vi "SPCCreateSetUpAsciiString.vi"(10 "Value":string[](array[string])=["5.0033574e-08"], 11 "Key":string[](array[string])=["SP_TAC_R,F,"]) -> (3 "SetUpAsciiString":string)   [LabVIEW 2019]
doc: "This VI demonstrates how specific parameters can be entered into an ASCII SetUp-block replacing their default values.\nProvide the Key up to and including the format specifier and trailing comma.\n\ninfo@becker-hickl.com"
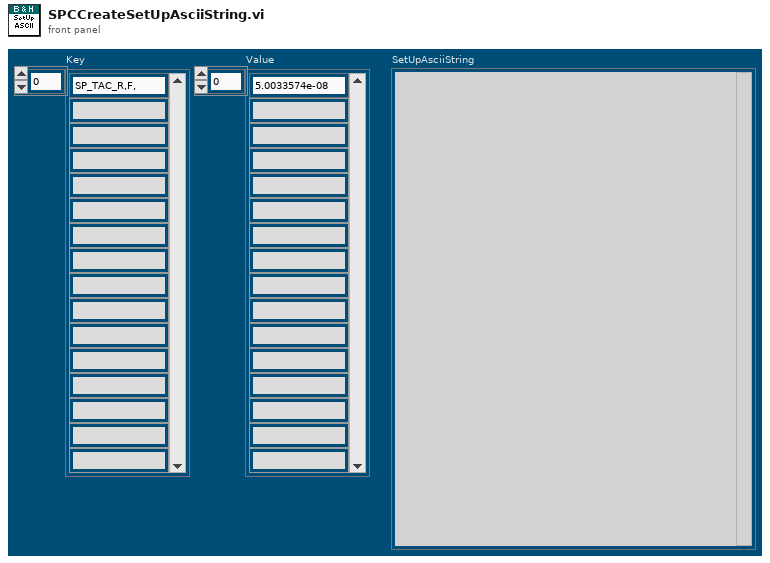
[diagram p1: front panel]
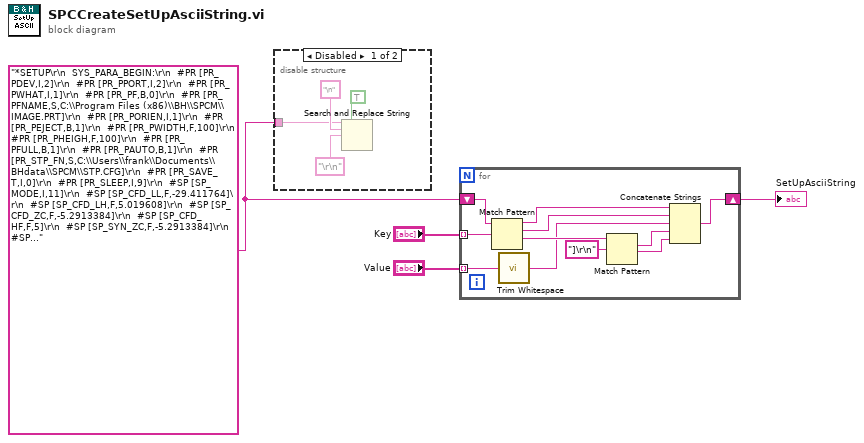
[diagram p0: block diagram]
diagram:
  w2 = "*SETUP\r\n  SYS_PARA_BEGIN:\r\n  #PR [PR_PDEV,I,2]\r\n  #PR [PR_PPORT,I,2]\r\n  #PR [PR_PWHAT,I,1]\r\n  #PR [PR_PF,B,0]\r\n  #PR [PR_PFNAME,S,C:\\Program Files (x86)\\BH\\SPCM\\IMAGE.PRT]\r\n  #PR [PR_PORIEN,I,1]\r\n  #PR [PR_PEJECT,B,1]\r\n  #PR [PR_PWIDTH,F,100]\r\n  #PR [PR_PHEIGH,F,100]\r\n  #PR [PR_PFULL,B,1]\r\n  #PR [PR_PAUTO,B,1]\r\n  #PR [PR_STP_FN,S,C:\\Users\\frank\\Documents\\BHdata\\SPCM\\STP.CFG]\r\n  #PR [PR_SAVE_T,I,0]\r\n  #PR [PR_SLEEP,I,9]\r\n  #SP [SP_MODE,I,11]\r\n  #SP [SP_CFD_LL,F,-29.411764]\r\n  #SP [SP_CFD_LH,F,5.019608]\r\n  #SP [SP_CFD_ZC,F,-5.2913384]\r\n  #SP [SP_CFD_HF,F,5]\r\n  #SP [SP_SYN_ZC,F,-5.2913384]\r\n  #SP [SP_SYN_FD,I,1]\r\n  #SP [SP_SYN_FQ,F,-50.980392]\r\n  #SP [SP_SYN_HF,F,4]\r\n  #SP [SP_TAC_R,F,5.0033574e-08]\r\n  #SP [SP_TAC_G,I,1]\r\n  #SP [SP_TAC_OF,F,0]\r\n  #SP [SP_TAC_LL,F,0]\r\n  #SP [SP_TAC_LH,F,100]\r\n  #SP [SP_TAC_TC,F,1.2215228e-11]\r\n  #SP [SP_TAC_TD,F,5.0033573e-09]\r\n  #SP [SP_ADC_RE,I,4096]\r\n  #SP [SP_EAL_DE,I,0]\r\n  #SP [SP_NCX,I,1]\r\n  #SP [SP_NCY,I,1]\r\n  #SP [SP_PAGE,I,1]\r\n  #SP [SP_COL_T,F,10]\r\n  #SP [SP_REP_T,F,10]\r\n  #SP [SP_DIS_T,F,1]\r\n  #SP [SP_REPEAT,B,0]\r\n  #SP [SP_STOPT,B,1]\r\n  #SP [SP_OVERFL,C,N]\r\n  #SP [SP_WL_STA,F,500]\r\n  #SP [SP_WL_STO,F,551.09998]\r\n  #SP [SP_WL_STE,F,0.1]\r\n  #SP [SP_EXTST,B,0]\r\n  #SP [SP_STEPS,I,64]\r\n  #SP [SP_OFFSET,F,0]\r\n  #SP [SP_YWIN_N,I,8]\r\n  #SP [SP_XWIN_N,I,8]\r\n  #SP [SP_TWIN_N,I,1]\r\n  #SP [SP_X_EQU,B,1]\r\n  #SP [SP_Y_EQU,B,1]\r\n  #SP [SP_T_EQU,B,1]\r\n  #SP [SP_DITH,I,128]\r\n  #SP [SP_EN_INT,B,0]\r\n  #SP [SP_INCR,I,1]\r\n  #SP [SP_DAES,B,0]\r\n  #SP [SP_SPE_FN,S,c:\\Users\\jannis\\Desktop\\SPC file example\\v1.spc]\r\n  #SP [SP_CYCLES,U,1]\r\n  #SP [SP_DAEC,B,1]\r\n  #SP [SP_MEM_BANK,I,0]\r\n  #SP [SP_DTCOMP,B,0]\r\n  #SP [SP_SCF,I,0]\r\n  #SP [SP_POL_L,I,0]\r\n  #SP [SP_POL_F,I,0]\r\n  #SP [SP_PIX,I,0]\r\n  #SP [SP_LDIV,I,0]\r\n  #SP [SP_ACCUM,B,0]\r\n  #SP [SP_ROUT,B,1792]\r\n  #SP [SP_TAC_EH,F,10]\r\n  #SP [SP_DLIM,I,10240000]\r\n  #SP [SP_PHOT_F,U,473956351]\r\n  #SP [SP_EN_DLIM,B,1]\r\n  #SP [SP_PH_BUF,I,65536]\r\n  #SP [SP_FLB_Y,I,1]\r\n  #SP [SP_FLB_X,I,1]\r\n  #SP [SP_BORD_U,I,1]\r\n  #SP [SP_BORD_L,I,1]\r\n  #SP [SP_POL_P,I,1]\r\n  #SP [SP_PIX_T,F,2.1e-05]\r\n  #SP [SP_PIX_CLK,I,1]\r\n  #SP [SP_TRIGGER,I,16]\r\n  #SP [SP_SCAN_X,I,1]\r\n  #SP [SP_SCAN_Y,I,1]\r\n  #SP [SP_SCAN_RX,I,1]\r\n  #SP [SP_SCAN_RY,I,1]\r\n  #SP [SP_FIF_TYP,I,0]\r\n  #SP [SP_EPX_DIV,I,1]\r\n  #SP [SP_MTCLK,I,0]\r\n  #SP [SP_ADD_SEL,I,0]\r\n  #SP [SP_SXWIN_N,I,1]\r\n  #SP [SP_SYWIN_N,I,1]\r\n  #SP [SP_SX_EQU,B,1]\r\n  #SP [SP_SY_EQU,B,1]\r\n  #SP [SP_ASAVE,I,34]\r\n  #SP [SP_ADC_ZOOM,I,0]\r\n  #SP [SP_FIF_FNO,I,1]\r\n  #SP [SP_FCYCLES,U,1]\r\n  #SP [SP_XY_GAIN,I,1]\r\n  #SP [SP_IMG_X,I,512]\r\n  #SP [SP_IMG_Y,I,512]\r\n  #SP [SP_IMG_RX,I,1]\r\n  #SP [SP_IMG_RY,I,1]\r\n  #SP [SP_MST_CLK,I,0]\r\n  #SP [SP_ADC_DE,I,0]\r\n  #SP [SP_DET_TYP,I,0]\r\n  #SP [SP_X_AXIS,I,0]\r\n  #SP [SP_CH_EN,I,4191231]\r\n  #SP [SP_CH_SL,I,16777215]\r\n  #SP [SP_CH_F1,I,0]\r\n  #SP [SP_CH_F2,I,136314880]\r\n  #DI [DI_SCALE,I,0]\r\n  #DI [DI_MAXCNT,L,2]\r\n  #DI [DI_LBLINE,L,1]\r\n  #DI [DI_BLINE,L,0]\r\n  #DI [DI_GRID,B,1]\r\n  #DI [DI_GCOL_F,I,14737632]\r\n  #DI [DI_GCOL_B,I,16777215]\r\n  #DI [DI_TRACE,I,0]\r\n  #DI [DI_BOD_C,I,32896]\r\n  #DI [DI_2DDIS,I,0]\r\n  #DI [DI_2DTRNO,I,1]\r\n  #DI [DI_3DOFFX,I,3]\r\n  #DI [DI_3DOFFY,I,1]\r\n  #DI [DI_3DINCX,I,0]\r\n  #DI [DI_3DCOL,I,0]\r\n  #DI [DI_3DMODE,I,2]\r\n  #DI [DI_YWIN,I,1]\r\n  #DI [DI_XWIN,I,1]\r\n  #DI [DI_TWIN,I,1]\r\n  #DI [DI_PSTYLE,I,1]\r\n  #DI [DI_PFREQ,I,1]\r\n  #DI [DI_CUR,B,0]\r\n  #DI [DI_RATE,B,1]\r\n  #DI [DI_2DC1,B,1]\r\n  #DI [DI_2DC2,B,1]\r\n  #DI [DI_2DC1C,I,10]\r\n  #DI [DI_2DC2C,I,13]\r\n  #DI [DI_2DC1S,I,0]\r\n  #DI [DI_2DC2S,I,0]\r\n  #DI [DI_3DC1C,I,12]\r\n  #DI [DI_3DC2C,I,14]\r\n  #DI [DI_SIZE,I,0]\r\n  #DI [DI_3DSTYL,I,1]\r\n  #DI [DI_INTCOL,I,1]\r\n  #DI [DI_INTPIX,I,1]\r\n  #DI [DI_COL_NO,I,2]\r\n  #DI [DI_COLMIN,I,0]\r\n  #DI [DI_COLMAX,I,16777215]\r\n  #DI [DI_COL2,I,16711680]\r\n  #DI [DI_COL3,I,255]\r\n  #DI [DI_COL4,I,16776960]\r\n  #DI [DI_COL5,I,65280]\r\n  #DI [DI_HICOL,I,16711680]\r\n  #DI [DI_XREV,B,0]\r\n  #DI [DI_YREV,B,0]\r\n  #DI [DI_DETAIL,B,1]\r\n  #DI [DI_SYWIN,I,1]\r\n  #DI [DI_SXWIN,I,1]\r\n  #DI [DI_ASCALE,I,1]\r\n  SYS_PARA_END:\r\n  TRACE_PARA_BEGIN:\r\n  #TR #0 [1,255,1,1,3,1,1,1]1,1,1]\r\n  #TR #1 [0,16711680,1,1,1,2,1,1]1,1,1]\r\n  #TR #2 [0,65280,1,1,1,3,1,1]1,1,1]\r\n  #TR #3 [0,44,1,1,1,4,1,1]1,1,1]\r\n  #TR #4 [0,16718521,1,1,1,1,1,1]1,1,1]\r\n  #TR #5 [0,16765696,1,1,1,1,1,1]1,1,1]\r\n  #TR #6 [0,22528,1,1,1,1,1,1]1,1,1]\r\n  #TR #7 [0,8684799,1,1,1,1,1,1]1,1,1]\r\n  #TR #8 [0,10374982,1,1,1,1,1,1]1,1,1]\r\n  #TR #9 [0,65473,1,1,1,1,1,1]1,1,1]\r\n  #TR #10 [0,33941,1,1,1,1,1,1]1,1,1]\r\n  #TR #11 [0,123,1,1,1,1,1,1]1,1,1]\r\n  #TR #12 [0,9818959,1,1,1,1,1,1]1,1,1]\r\n  #TR #13 [0,16162524,1,1,1,1,1,1]1,1,1]\r\n  #TR #14 [0,13832959,1,1,1,1,1,1]1,1,1]\r\n  #TR #15 [0,8067690,1,1,1,1,1,1]1,1,1]\r\n  TRACE_PARA_END:\r\n  WIND_PARA_BEGIN:\r\n  #WI #0 *NO *0 [0,0]\r\n  #WI #0 *NO *1 [1,1]\r\n  #WI #0 *NO *2 [2,2]\r\n  #WI #0 *NO *3 [3,3]\r\n  #WI #0 *NO *4 [4,4]\r\n  #WI #0 *NO *5 [5,5]\r\n  #WI #0 *NO *6 [6,6]\r\n  #WI #0 *NO *7 [7,7]\r\n  #WI #1 *NO *0 [0,0]\r\n  #WI #1 *NO *1 [0,0]\r\n  #WI #1 *NO *2 [0,0]\r\n  #WI #1 *NO *3 [0,0]\r\n  #WI #1 *NO *4 [0,0]\r\n  #WI #1 *NO *5 [0,0]\r\n  #WI #1 *NO *6 [0,0]\r\n  #WI #1 *NO *7 [0,0]\r\n  #WI #2 *NO *0 [0,4095]\r\n  #WI #3 *NO *0 [0,0]\r\n  #WI #4 *NO *0 [0,0]\r\n  WIND_PARA_END:\r\n*END" ("result string")
  n1 = disable-structure shown="Disabled" {
    disable-tunnel: w2 -> [w5 _]
    frame Disabled {
      n2 = Search and Replace String(replace all?=TRUE ("replace all? (F)"), input string=w5, search string="\n" ("regular expression"), replace string="\r\n" ("regular expression")) -> ()  [unwired: 4 in, 4 out]
    }
    frame Enabled {
    }
  }
  n3 = for {
    tunnel: "Key" -> [w17] mode=indexing
    shift-right: [w15] -> w3
    shift-left: w2 -> [w16]
    tunnel: "Value" -> [w10] mode=indexing
    n4 = Match Pattern(string=w16, regular expression=w17) -> (before substring=w14:string, match substring=w13:string, after substring=w19:string)  [unwired: 1 in, 1 out]
    n5 = call <vilib>:"Trim Whitespace.vi"("string"=w10) -> ("trimmed string"=w9:string)  [unwired: 1 in]
    n6 = Match Pattern(string=w19, regular expression="]\r\n") -> (match substring=w12:string, after substring=w11:string)  [unwired: 1 in, 2 out]
    n7 = Concatenate Strings(w14, w13, w9, w12, w11) -> (w15:string)
  }
  "SetUpAsciiString" <- w3
